vi "AutoBin.vi"(10 "strength":dbl, 11 "State Wire OUT in":T1 {"Sorted Sweep Info"."Sorted scan parameters"."?"."Rate" format="%.2f"; "Sorted Sweep Info"."Sorted scan parameters"."?"."Step" format="%#_6p"; "Sorted Sweep Info"."Sorted scan parameters"."?"."End" format="%#_6p"; "Sorted Sweep Info"."Sorted scan parameters"."?"."Start" format="%#_6p"; "X Step Info"."X Step" format="%#_6p"; "X Step Info"."X High" format="%#_6p"; "X Step Info"."X Low" format="%#_6p"}) -> (1 "auto min":dbl, 2 "auto max":dbl, 3 "State Wire OUT in 2":T1 {"Sorted Sweep Info"."Sorted scan parameters"."?"."Rate" format="%.2f"; "Sorted Sweep Info"."Sorted scan parameters"."?"."Step" format="%#_6p"; "Sorted Sweep Info"."Sorted scan parameters"."?"."End" format="%#_6p"; "Sorted Sweep Info"."Sorted scan parameters"."?"."Start" format="%#_6p"; "X Step Info"."X Step" format="%#_6p"; "X Step Info"."X High" format="%#_6p"; "X Step Info"."X Low" format="%#_6p"})   [LabVIEW 2016]
uses:
  ZDataVIS_StateWire.ctl
  <vilib>/Utility/miscctls.llb/LVPointDoubleTypeDef.ctl
  <userlib>/_OpenG.lib/dictionary/dictionary.llb/Dictionary Object RefNum__ogtk.ctl
  <userlib>/_OpenG.lib/dictionary/dictionary.llb/Dictionary Object RefNum - Enum__ogtk.ctl
  <userlib>/LevyLab/Transport/SweepControl/Typedefs/ScanControl.ctl
  <userlib>/LevyLab/Transport/SweepControl/Typedefs/Cluster - ScanControl.ctl
  <userlib>/LevyLab/Transport/SweepControl/Typedefs/Enum - Priority.ctl
  <userlib>/LevyLab/Transport/SweepControl/Typedefs/Enum - Action.ctl
  <userlib>/LevyLab/Transport/SweepControl/Typedefs/ScanParamters.ctl
  <userlib>/LevyLab/Transport/SweepControl/Typedefs/Cluster - ScanParamters.ctl
  <userlib>/LevyLab/Transport/SweepControl/Typedefs/Enum - Experiments.ctl
  <userlib>/LevyLab/Transport/SweepControl/SweepControl.lvclass
panel:
  # "cursor x"
  # "cursor y"
  # "cursor x"
  # "cursor y"
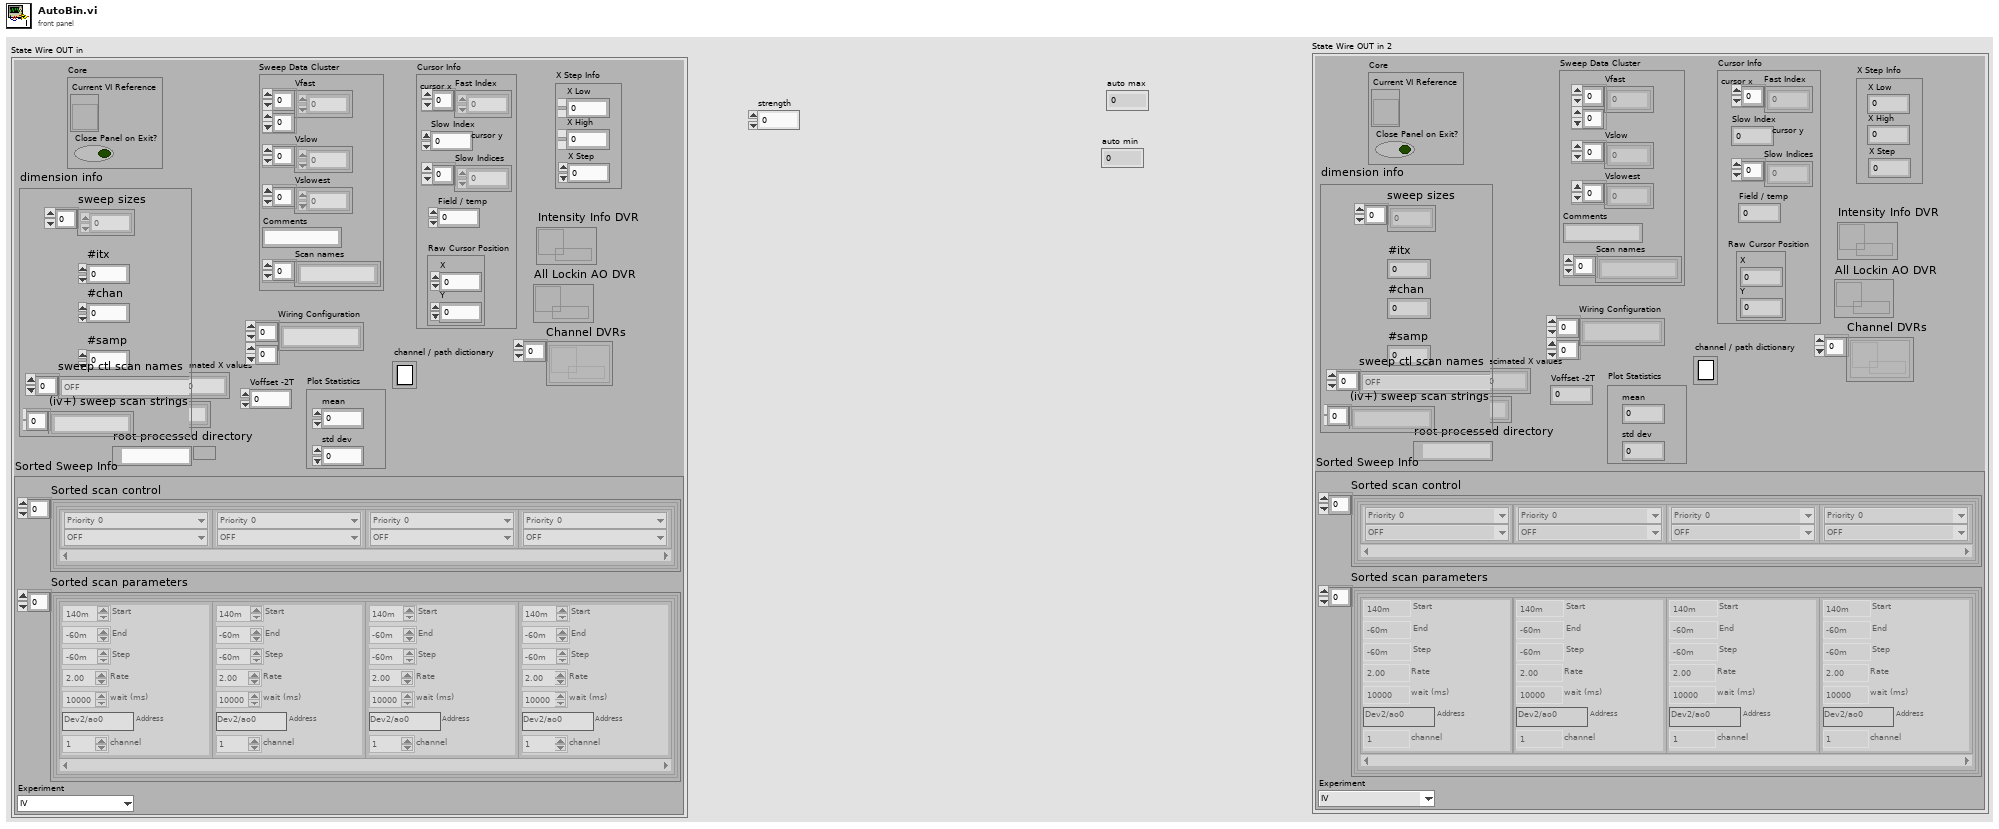
[diagram p1: front panel]
types:
  T1 = typedef "ZDataVIS_StateWire.ctl" = cluster{"Core":cluster{"Current VI Reference":refnum<vi>, "Close Panel on Exit?":bool}, "Channel DVRs":refnum<data-value>[], "Sweep Data Cluster":cluster{"Vfast":dbl[][], "Vslow":dbl[], "Vslowest":dbl[], "Comments":string, "Scan names":string[]}, "Cursor Info":cluster{"Fast Index":dbl[], "Slow Index":dbl, "Slow Indices":dbl[], "Raw Cursor Position":T2, "Field / temp":i32}, "Scan names":string[], "Decimated X values":dbl[], "X Step Info":cluster{"X Low":dbl, "X High":dbl, "X Step":dbl}, "Voffset -2T":dbl, "Wiring Configuration ":string[][], "Intensity Info DVR":refnum<data-value>, "Object RefNum":T3, "All Lockin AO DVR":refnum<data-value>, "root processed directory":path, "Sorted Sweep Info":cluster{"Sorted scan control":cluster{T4}[], "Sorted scan parameters":cluster{T8}[], "Experiment":T10}, "dimension info":cluster{"sweep sizes":i32[], "#itx":i32, "#chan":i32, "#samp":i32, "sweep ctl scan names":T7[], "(iv+) sweep scan strings":string[]}, "Plot Statistics":cluster{"mean":dbl, "std dev":dbl}}
  T2 = typedef "LVPointDoubleTypeDef.ctl" = cluster{"X":dbl, "Y":dbl}
  T3 = typedef "Dictionary Object RefNum__ogtk.ctl" = refnum<k1>
  T4 = typedef "SweepControl.lvclass/ScanControl.ctl" = T5[]
  T5 = typedef "SweepControl.lvclass/Cluster - ScanControl.ctl" = cluster{"Priority":T6, "Scan name":T7}
  T6 = typedef "SweepControl.lvclass/Enum - Priority.ctl" = enum16{"Priority 0", "Priority 1", "Priority 2", "Priority 3", "Priority 4", "Priority 5"}
  T7 = typedef "SweepControl.lvclass/Enum - Action.ctl" = enum16{"OFF", "DSA_Vamp", "DSA_freq", "DSA_Vsg1", "DSA_Vsg2", "DSA_Vsg3", "DAQ_Vbg", "B_Field", "Humidity", "Temp", "MW_freq1", "MW_freq2", "MW_amplitude1", "MW_amplitude2"}
  T8 = typedef "SweepControl.lvclass/ScanParamters.ctl" = T9[]
  T9 = typedef "SweepControl.lvclass/Cluster - ScanParamters.ctl" = cluster{"Start":dbl, "End":dbl, "Step":dbl, "Rate":dbl, "wait (ms)":u32, "Address":string, "channel":i32}
  T10 = typedef "SweepControl.lvclass/Enum - Experiments.ctl" = enum16{"IV", "Lockin_time", "Lockin_Vsg", "Lockin (experimental)", "Lockin_Vsg_JKISM"}
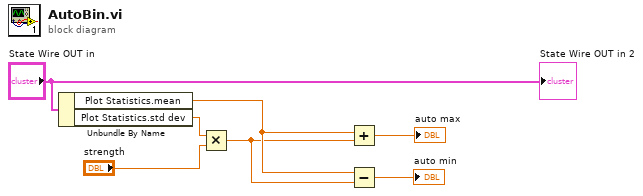
[diagram p0: block diagram]
diagram:
  n1 = Unbundle By Name("State Wire OUT in") -> ("Plot Statistics.mean"=w2:dbl, "Plot Statistics.std dev"=w6:dbl)
  n2 = Multiply(x=w6, y="strength") -> (x*y=w1:dbl)
  n3 = Add(x=w2, y=w1) -> (x+y=→"auto max":dbl)
  n4 = Subtract(x=w2, y=w1) -> (x-y=→"auto min":dbl)
  "State Wire OUT in 2" <- "State Wire OUT in"
